vi "3xMonitor.vi"   [LabVIEW 2016]
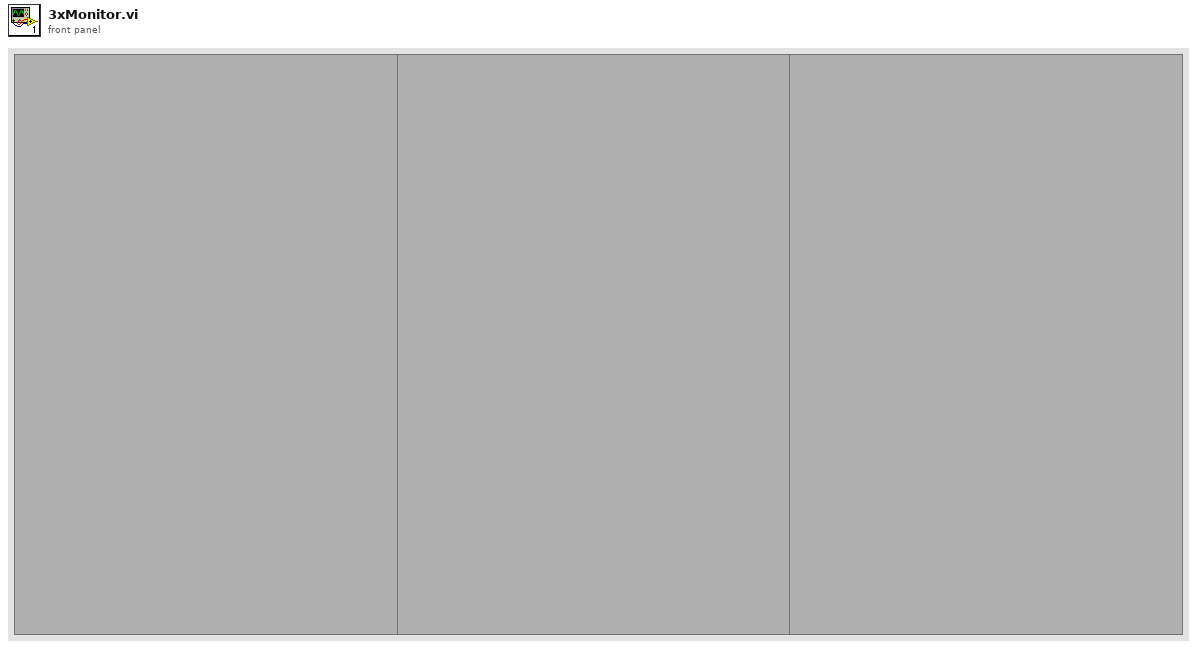
[diagram p1: front panel]
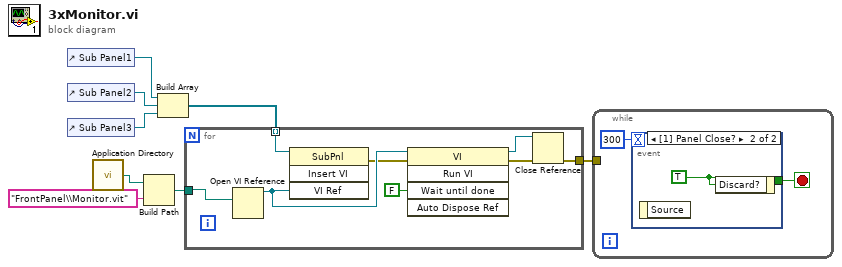
[diagram p0: block diagram]
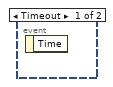
[diagram p2: hidden frame]
diagram:
  n1 = control-ref of="Sub Panel1"() -> (w8:refnum<vi>)
  n2 = control-ref of="Sub Panel2"() -> (w7:refnum<vi>)
  n3 = control-ref of="Sub Panel3"() -> (w6:refnum<vi>)
  n4 = call <vilib>:"Application Directory.vi"() -> ("Application Directory"=w5:path)
  n5 = Build Path(base path=w5, name or relative path="FrontPanel\\Monitor.vit") -> (appended path=w4:path)
  n6 = Build Array(w8, w7, w6) -> (w1:refnum<vi>[])
  n7 = for {
    tunnel: w4 -> [w12]
    tunnel: w1 -> [w16] mode=indexing
    tunnel: [w9] -> w2
    n8 = Open VI Reference(vi path=w12) -> (vi reference=w15:refnum<vi>)  [unwired: 5 in, 1 out]
    n9 = invoke on="Invoke Node" class="SubPnl" method="Insert VI"(reference=w16, "VI Ref"=w15) -> (error out=w14:errorcluster)  [unwired: 2 in, 3 out]
    n10 = invoke class="VI" method="Run VI"(reference=w15, error in=w14, "Wait until done"=FALSE ("Wait Until Done")) -> (reference out=w11:refnum<vi>, error out=w10:errorcluster)  [unwired: 2 in, 3 out]
    n11 = Close Reference(reference=w11, error in (no error)=w10) -> (error out=w9:errorcluster)
  }
  n12 = while {
    tunnel: w2 -> [_]
    stop <- w18 stop-if-true
    n13 = event shown="[1] Panel Close?" {
      selector: _ -> [_ _]
      dyn-events: _ -> [_ _]
      timeout: 300 -> [_ _]
      tunnel: [_ w19] -> w18
      event Timeout {
        n14 = event-data() -> ()  [unwired: 1 in, 1 out]
      }
      event Panel Close? {
        w19 = TRUE ("stop")
        n15 = event-data() -> ()  [unwired: 1 in, 1 out]
        n16 = event-data("Discard?"=w19) -> ()  [unwired: 1 in, 1 out]
      }
    }
  }
